vi "Queues FGV.vi"(7 "Enum":T2, 8 "error in (no error)":errorcluster) -> (0 "error out":errorcluster, 3 "Inner Process Queues Cluester":T1)   [LabVIEW 2023, in "Innes Process Communication.lvlib"]
uses:
  Innes Process Communication.lvlib
  States Queues FGV.ctl
  Inner Proccess Cluster Queues.ctl
  Message.ctl
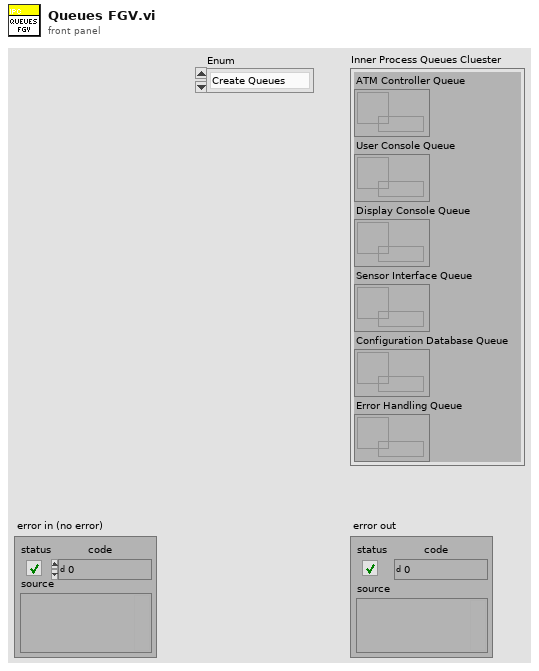
[diagram p1: front panel]
types:
  T1 = typedef "Innes Process Communication.lvlib/Inner Proccess Cluster Queues.ctl" = cluster{"ATM Controller Queue":refnum<queue>, "User Console Queue":refnum<queue>, "Display Console Queue":refnum<queue>, "Sensor Interface Queue":refnum<queue>, "Configuration Database Queue":refnum<queue>, "Error Handling Queue":refnum<queue>}
  T2 = typedef "Innes Process Communication.lvlib/States Queues FGV.ctl" = enum16{"Create Queues", "Get Queues", "Destroy Queues"}
  T3 = typedef "Innes Process Communication.lvlib/Message.ctl" = cluster{"Command":string, "Data":variant}
  T4 = cluster{"Display Console Queue":refnum<queue>, "ATM Controller Queue":refnum<queue>, "User Console Queue":refnum<queue>, "Sensor Interface Queue":refnum<queue>, "Configuration Database Queue":refnum<queue>, "Error Handling Queue":refnum<queue>}
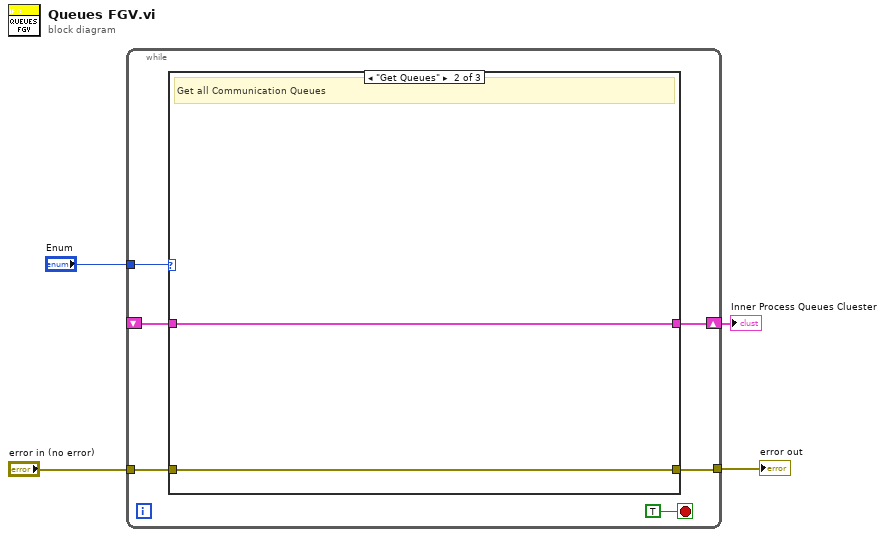
[diagram p0: block diagram]
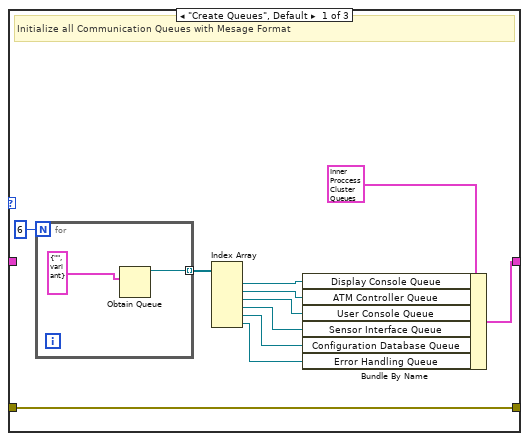
[diagram p2: hidden frame]
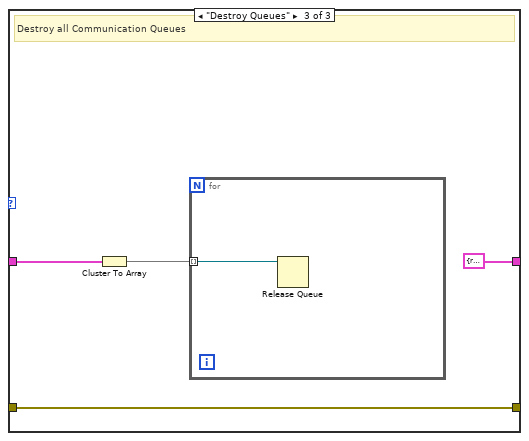
[diagram p3: hidden frame]
diagram:
  n1 = while {
    shift-right: [w10] -> w1
    shift-left: _ -> [w7]
    tunnel: "Enum" -> [w8]
    tunnel: [w6] -> w2
    tunnel: "error in (no error)" -> [w5]
    stop <- TRUE stop-if-true
    n2 = case shown="\"Get Queues\"" w8 {
      tunnel: [w20 w25 T4 {"Display Console Queue"=refnum, "ATM Controller Queue"=refnum, "User Console Queue"=refnum, "Sensor Interface Queue"=refnum, "Configuration Database Queue"=refnum, "Error Handling Queue"=refnum} ("Inner Process Queues Cluester")] -> w10
      tunnel: w7 -> [_ w25 w29]
      tunnel: [w18 w24 w26] -> w6
      tunnel: w5 -> [w18 w24 w26]
      frame "Create Queues", Default {
        # "Initialize all Communication Queues with Mesage Format"
        n3 = for {
          N: 6 -> [_]
          tunnel: [w23] -> w21 mode=indexing
          n4 = Obtain Queue(element data type=T3 {"Command"="", "Data"=variant} ("Message")) -> (queue out=w23:refnum<queue>)  [unwired: 4 in, 2 out]
        }
        n5 = Index Array(array=w21) -> (element #1=w16:refnum<queue>, element #2=w15:refnum<queue>, element #3=w14:refnum<queue>, element #4=w13:refnum<queue>, element #5=w12:refnum<queue>, element #6=w11:refnum<queue>)  [unwired: 6 in]
        n6 = Bundle By Name(cluster=T1 {"ATM Controller Queue"=refnum, "User Console Queue"=refnum, "Display Console Queue"=refnum, "Sensor Interface Queue"=refnum, "Configuration Database Queue"=refnum, "Error Handling Queue"=refnum} ("Inner Process Queues Cluester"), "Display Console Queue"=w16, "ATM Controller Queue"=w15, "User Console Queue"=w14, "Sensor Interface Queue"=w13, "Configuration Database Queue"=w12, "Error Handling Queue"=w11) -> (w20:T1)
      }
      frame "Get Queues" {
        # "Get all Communication Queues"
      }
      frame "Destroy Queues" {
        # "Destroy all Communication Queues"
        n7 = Cluster To Array(cluster=w29) -> (array=w28:refnum<queue>[])
        n8 = for {
          tunnel: w28 -> [w30] mode=indexing
          n9 = Release Queue(queue=w30) -> ()  [unwired: 2 in, 3 out]
        }
      }
    }
  }
  "error out" <- w2
  "Inner Process Queues Cluester" <- w1
